vi "Primative_Duty_Cycle.vi"(3 "Input power":dbl) -> (0 "Duty cycle acheived":dbl, 1 "Mins on":i32[](array[numeric]))   [LabVIEW 2012]
panel:
  out "size(s)":i32
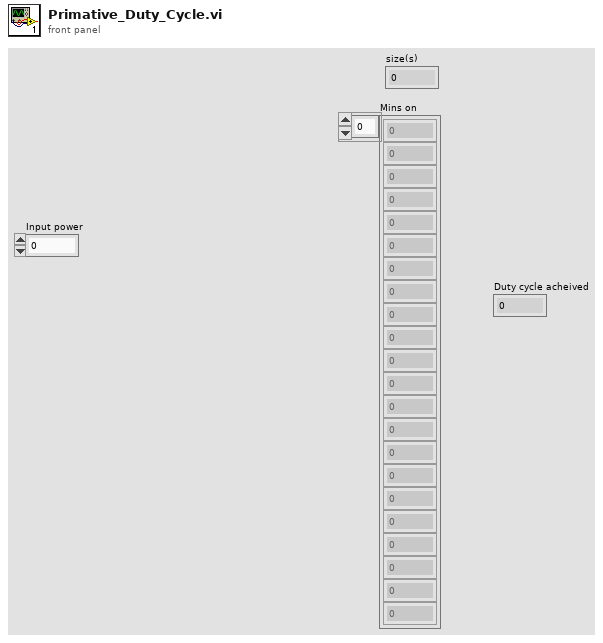
[diagram p1: front panel]
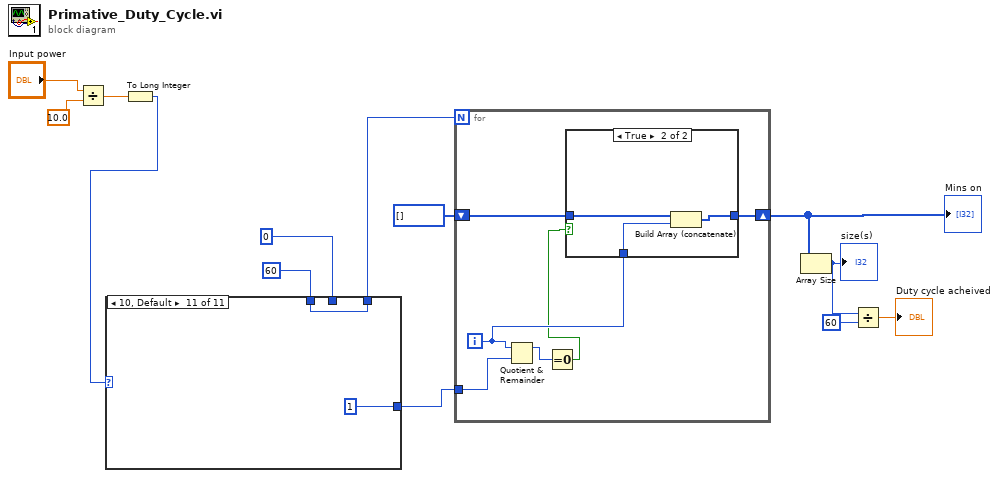
[diagram p0: block diagram]
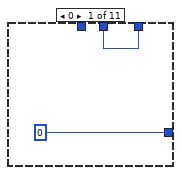
[diagram p2: hidden frame]
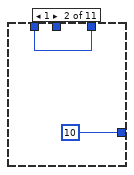
[diagram p3: hidden frame]
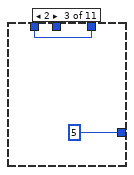
[diagram p4: hidden frame]
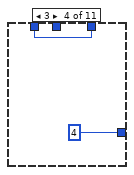
[diagram p5: hidden frame]
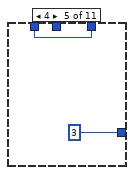
[diagram p6: hidden frame]
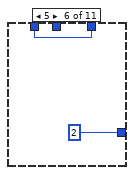
[diagram p7: hidden frame]
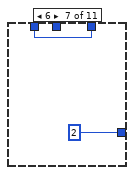
[diagram p8: hidden frame]
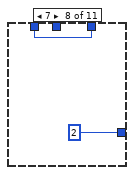
[diagram p9: hidden frame]
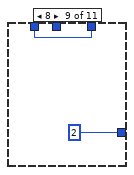
[diagram p10: hidden frame]
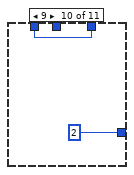
[diagram p11: hidden frame]
diagram:
  n1 = Divide(x="Input power", y=10.0) -> (x/y=w6:dbl)
  n2 = To Long Integer(number=w6) -> (32bit integer=w5:i32)
  n3 = case shown="10, Default" w5 {
    tunnel: [0 10 5 4 3 2 2 2 2 2 1] -> w4
    tunnel: [w14 w16 w18 w20 w22 w24 w26 w28 w30 w32 w34] -> w3
    tunnel: 0 -> [w14 _ _ _ _ _ _ _ _ _ _]
    tunnel: 60 -> [_ w16 w18 w20 w22 w24 w26 w28 w30 w32 w34]
    frame 0 {
    }
    frame 1 {
    }
    frame 2 {
    }
    frame 3 {
    }
    frame 4 {
    }
    frame 5 {
    }
    frame 6 {
    }
    frame 7 {
    }
    frame 8 {
    }
    frame 9 {
    }
    frame 10, Default {
    }
  }
  n4 = for {
    N: w3 -> [_]
    shift-right: [w39] -> w10
    shift-left: i32[] [] -> [w40]
    tunnel: w4 -> [w38]
    i -> [w41]
    n5 = Quotient & Remainder(x=w41, y=w38) -> (x-y*floor(x/y)=w37:i32)  [unwired: 1 out]
    n6 = Equal To 0?(x=w37) -> (x = 0?=w36:bool)
    n7 = case shown="True" w36 {
      tunnel: w41 -> [_ w43]
      tunnel: w40 -> [w42 w45]
      tunnel: [w42 w44] -> w39
      frame False {
      }
      frame True {
        n8 = Build Array (concatenate)(w45, w43) -> (w44:i32[])
      }
    }
  }
  "Mins on" <- w10
  n9 = Array Size(array=w10) -> (size(s)=w9:i32)
  "size(s)" <- w9
  n10 = Divide(x=w9, y=60) -> (x/y=→"Duty cycle acheived":dbl)
